vi "Write Child Actor Attributes.vi"(7 "Actor in":refnum<class "Actor.lvclass">, 10 "Child Actor Attributes":refnum<data-value>) -> (5 "Actor out":refnum<class "Actor.lvclass">)   [LabVIEW 2020, in "jettl.lvlib"]
uses:
  jettl.lvlib
  Msg/Msg.lvclass
  Actor/Actor.lvclass
  Refs/Refs.lvclass
  Msg Input/Msg Input.lvclass
  Msg Output/Msg Output.lvclass
  Msgs.ctl
  Unified Layer.ctl
  Actor Attributes.ctl
  Child Actor Attributes.ctl
  Relation.ctl
  Teller.ctl
  Msg Attributes.ctl
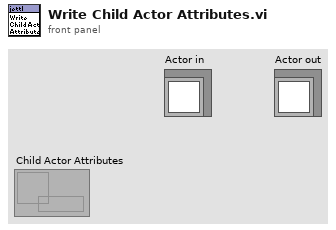
[diagram p1: front panel]
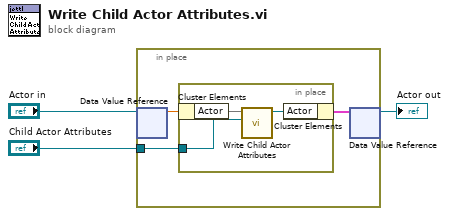
[diagram p0: block diagram]
diagram:
  n1 = in-place {
    in-place-border: "Child Actor Attributes" -> [w4]
    n2 = in-place-dvr #1("Actor in") -> (w6:dbl)  [unwired: 1 out]
    n3 = in-place {
      in-place-border: w4 -> [w7]
      n4 = in-place-cluster #2(w6) -> ("Actor"=w9)
      n5 = call-dynamic "Write Child Actor Attributes.vi"("Child Actor Attributes"=w7, "Actor in"=w9) -> ("Actor out"=w8:refnum<class "Actor.lvclass">)  [unwired: 9 in]
      n6 = in-place-cluster #2("Actor"=w8) -> (w5:cluster{})
    }
    n7 = in-place-dvr #1(w5) -> (→"Actor out":refnum<data-value>)  [unwired: 1 out]
  }
